vi "PhaseSpace.vi"() -> ()   [LabVIEW 2018]
uses:
  <vilib>/Platform/TimedLoop/XDataNode/timing_clust.ctl
  <vilib>/Platform/TimedLoop/XDataNode/nitl_modes.ctl
  <vilib>/Platform/TimedLoop/XDataNode/wakeup.ctl
  Global Variables/Sensor_Impluse.vi
  Global Variables/Sensor_Force.vi
  <vilib>/express/express shared/transition.llb/Dynamic To Waveform Array.vi
  <vilib>/express/express signal manip/GetorSetDDTAttributes/Set DDT Attributes/SetT0.vi
  <vilib>/express/express shared/transition.llb/Waveform Array To Dynamic.vi
  <vilib>/Platform/TimedLoop/XDataNode/XDataNode.xnode
  <vilib>/express/express signal manip/GetorSetDDTAttributes/Set DDT Attributes/Set DDT Properties.xnode
  <vilib>/Platform/TimedLoop/XDataNode/XDNodeRunTimeDep.lvlib
  <vilib>/Analysis/NI_AALBase.lvlib
  <vilib>/Analysis/NI_AALPro.lvlib
  <vilib>/Analysis/coordinate.llb/Euler Rotation Order.ctl
  <vilib>/Analysis/baseanly.llb/Real A x B.vi
  <vilib>/Analysis/baseanly.llb/A x Vector.vi
panel:
  out "A x Vector":dbl[](array[numeric]) format="%.2f"
  out "Root canal 2":dbl[](array[numeric])
  out "Count":u32
  out "element":i32
  in  "Record":bool
  in  "Save?":bool
  out "Frame 2":string
  out "LED ID":i32
  out "Y position (mm) 8":string
  out "X position (mm) 8":string
  out "Z position (mm) 8":string
  out "_LED 1":dbl[](array[numeric])
  out "Y position (mm) 9":string
  out "X position (mm) 9":string
  out "Z position (mm) 9":string
  out "_LED 2":dbl[](array[numeric])
  out "Y position (mm) 10":string
  out "X position (mm) 10":string
  out "Z position (mm) 10":string
  out "_LED3":dbl[](array[numeric])
  out "Z position (mm) 11":string
  out "Y position (mm) 11":string
  out "X position (mm) 11":string
  out "_LED4":dbl[](array[numeric])
  in  "TrackingLED 3":i32=15
  in  "TrackingLED 2":i32=15
  in  "TrackingLED 1":i32=15
  in  "Server IP address 2":string="192.168.50.40"
  in  "stop":bool
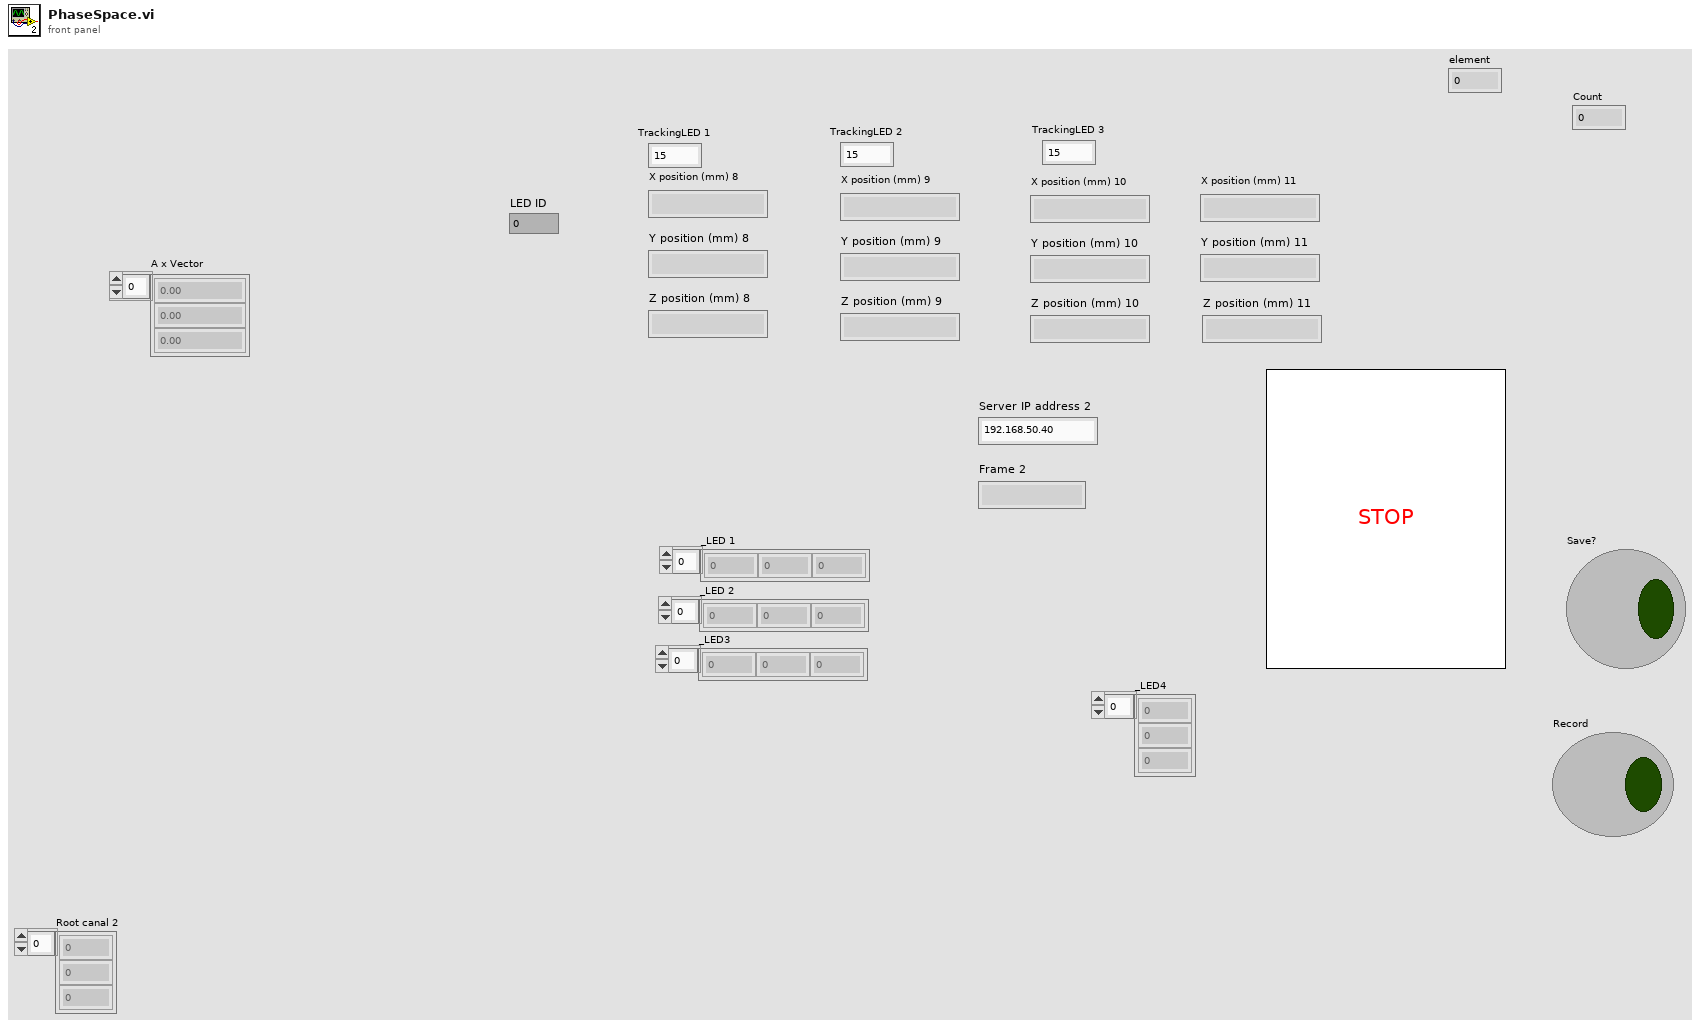
[diagram p1: front panel]
types:
  T1 = typedef "XDNodeRunTimeDep.lvlib/timing_clust.ctl" = cluster{"Expected End [f-1]":u64, "Actual End [f-1]":u64, "Finished Late? [f-1]":bool, "Expected End [i-1]":u64, "Actual End [i-1]":u64, "Finished Late? [i-1]":bool, "Expected Start [i]":u64, "Actual Start [i]":u64, "Expected Start [f]":u64, "Actual Start [f]":u64, "Source Name":string, "Structure Name":string, "Period":i64, "Deadline":i64, "Offset":i64, "Start":i64, "Priority":i32, "Timeout":i32, "Mode":T2, "Wakeup Reason":T3, "Error":errorcluster, "Source Type":string, "Secondary Source Type":string, "Global End Time":u64, "Global Start Time":u64, "Frame Duration":u64, "Iteration Duration":u64, "Assigned CPU":i32, "I/O Scan Engine Mode":u32}
  T2 = typedef "XDNodeRunTimeDep.lvlib/nitl_modes.ctl" = enum32{"No Change", "Process missed periods, maintain original phase", "Discard missed periods, maintain original phase", "Process missed periods, ignore original phase", "Discard missed periods, ignore original phase"}
  T3 = typedef "XDNodeRunTimeDep.lvlib/wakeup.ctl" = enum32{"Normal", "Aborted", "Asynchronous wakeup", "Timing source error", "Timed loop error", "Timeout"}
  T4 = typedef "NI_AALPro.lvlib/Euler Rotation Order.ctl" = u16
  T5 = typedef "NI_Matrix.lvlib/RealMatrix.ctl" = dbl[][]
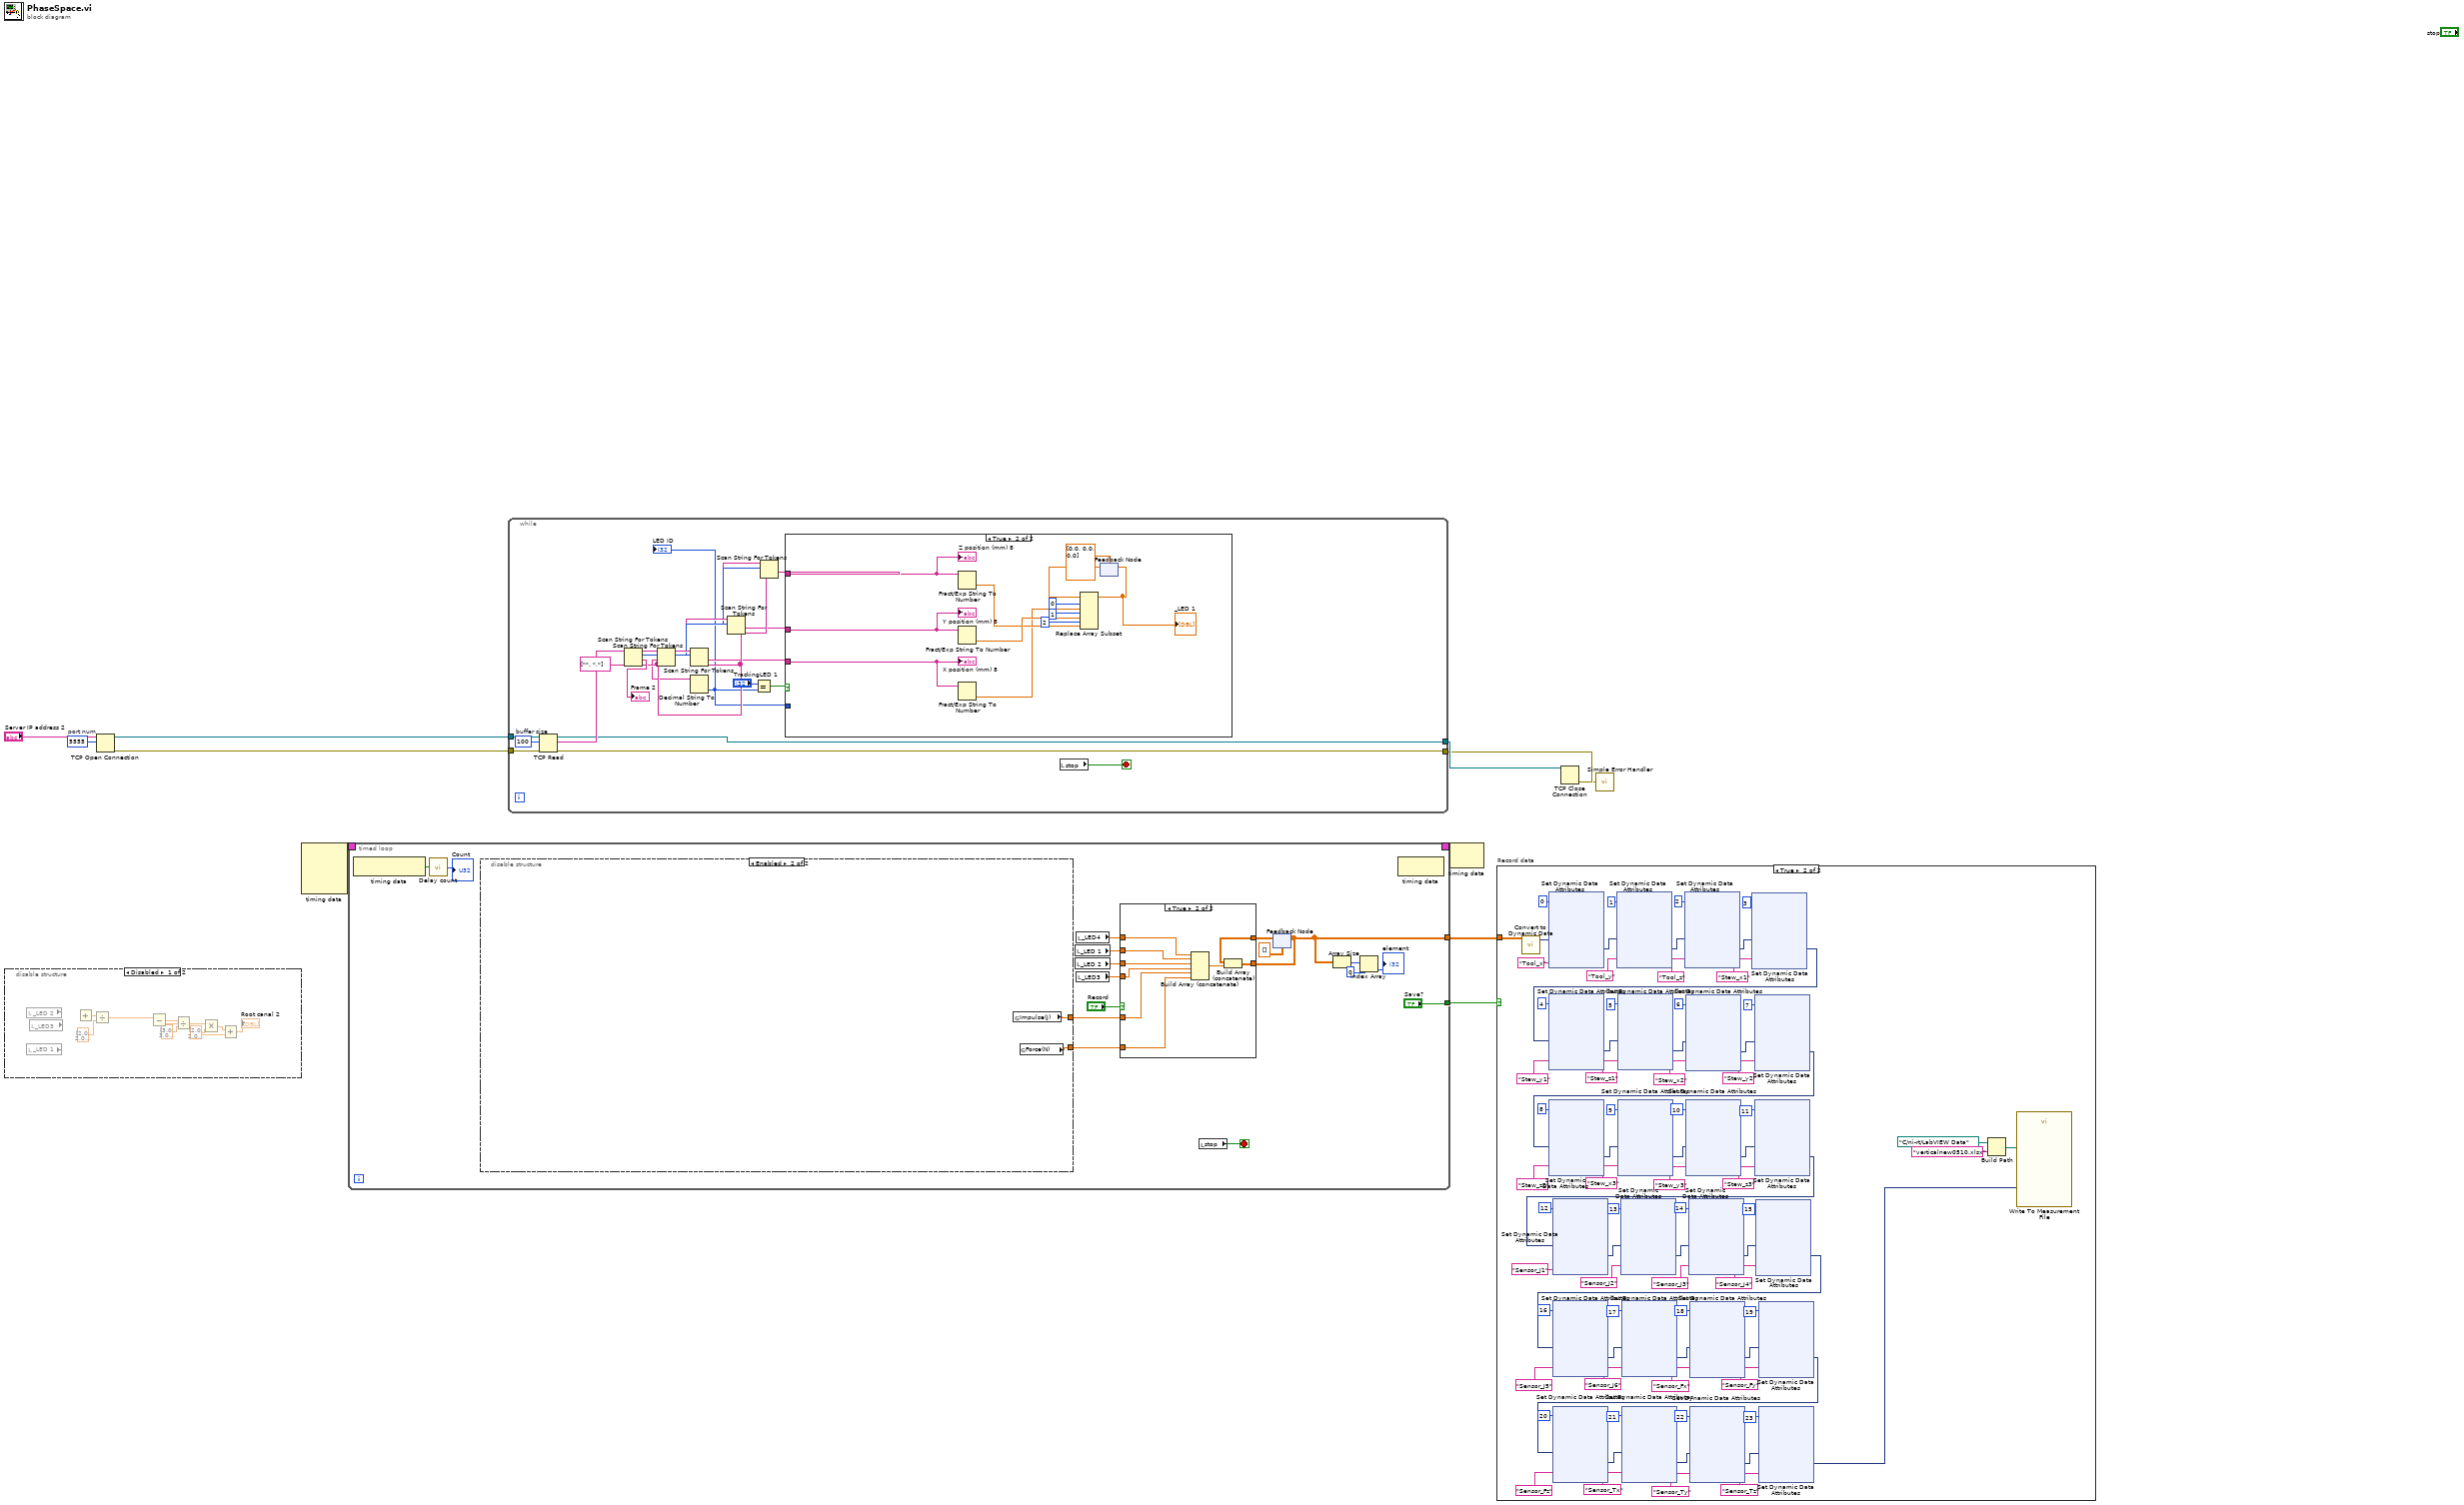
[diagram p0: block diagram]
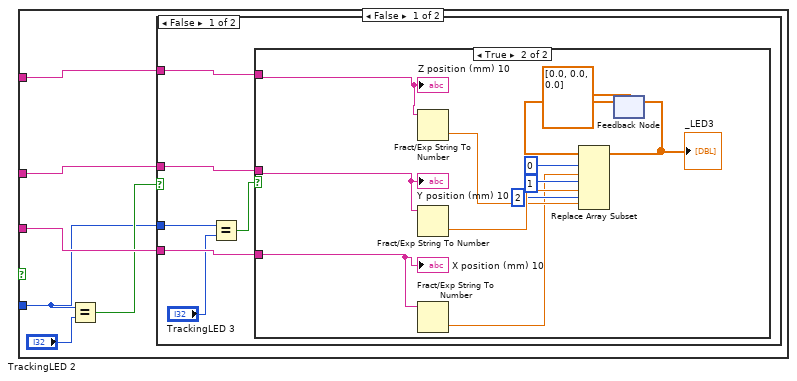
[diagram p3: hidden frame]
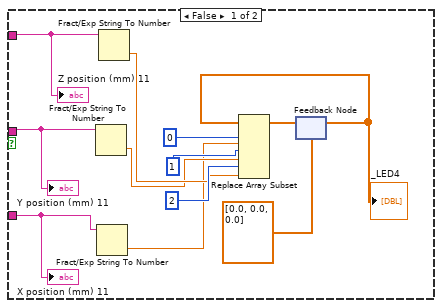
[diagram p4: hidden frame]
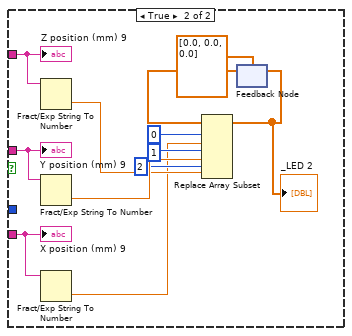
[diagram p5: hidden frame]
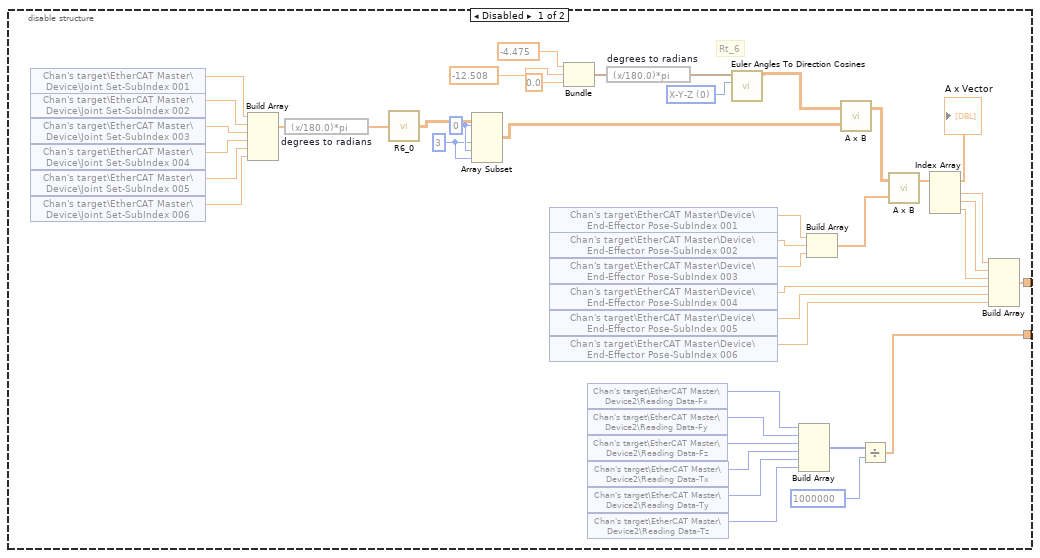
[diagram p6: hidden frame]
diagram:
  w9 = 5555  # port num
  n1 = disable-structure shown="Disabled" {
    frame Disabled {
      n2 = local read "_LED 2"() -> (w13:dbl[])
      n3 = local read "_LED 1"() -> (w12:dbl[])
      n4 = local read "_LED3"() -> ()  [unwired: 1 out]
      n5 = Add() -> (x+y=w22:dbl)  [unwired: 2 in]
      n6 = Divide(x=w22, y=dbl[] [2.0, 2.0, 2.0]) -> (x/y=w21:dbl[])
      n7 = Subtract(x=w21, y=w17) -> (x-y=w19:dbl[])
      n8 = Divide(x=w19, y=dbl[] [3.0, 3.0, 3.0]) -> (x/y=w20:dbl[])
      n9 = Multiply(x=w20, y=dbl[] [2.0, 2.0, 2.0]) -> (x*y=w18:dbl[])
      n10 = Add(x=w18) -> (y=w17:dbl[], x+y=→"Root canal 2":dbl[])
    }
    frame Enabled {
    }
  }
  n11 = TCP Open Connection(address="Server IP address 2", remote port or service name=w9) -> (connection ID=w10:refnum<k5>, error out=w11:errorcluster)  [unwired: 3 in]
  n12 = node-c288() -> (w4:T1)  [unwired: 4 in]
  n13 = timed-loop {
    timing: w4 -> [_]
    timing-out: [_] -> w3
    tunnel: ["Save?"] -> w2
    tunnel: [w35] -> w1
    stop <- w31 stop-if-true
    n14 = node-c288() -> (w30:bool)  [unwired: 1 in]
    n15 = call "Delay count.vi"("Finished Late? [i-1]"=w30) -> ("Count"=→"Count":u32)
    n16 = disable-structure shown="Enabled" {
      disable-tunnel: [w70 w83] -> w27
      disable-tunnel: [w69 w82] -> w26
      frame Disabled {
        w45 = 0 ("row 1")
        w44 = 3 ("row N")
        w52 = T4 0 items=["X-Y-Z", "X-Z-Y", "Y-X-Z", "Y-Z-X", "Z-X-Y", "Z-Y-X", "X-Y-X", "X-Z-X", "Y-X-Y", "Y-Z-Y", "Z-X-Z", "Z-Y-Z"] ("rotation order")
        # "Rt_6"
        n17 = shared-variable "Chan's target\\EtherCAT Master\\Device\\Joint Set-SubIndex 001"() -> (w68:sgl)  [unwired: 1 in, 1 out]
        n18 = shared-variable "Chan's target\\EtherCAT Master\\Device\\Joint Set-SubIndex 002"() -> (w67:sgl)  [unwired: 1 in, 1 out]
        n19 = shared-variable "Chan's target\\EtherCAT Master\\Device\\Joint Set-SubIndex 003"() -> (w66:sgl)  [unwired: 1 in, 1 out]
        n20 = shared-variable "Chan's target\\EtherCAT Master\\Device\\Joint Set-SubIndex 004"() -> (w65:sgl)  [unwired: 1 in, 1 out]
        n21 = shared-variable "Chan's target\\EtherCAT Master\\Device\\Joint Set-SubIndex 005"() -> (w64:sgl)  [unwired: 1 in, 1 out]
        n22 = shared-variable "Chan's target\\EtherCAT Master\\Device\\Joint Set-SubIndex 006"() -> (w63:sgl)  [unwired: 1 in, 1 out]
        n23 = Build Array(w68, w67, w66, w65, w64, w63) -> (w42:sgl[])
        n24 = expression code="(x/180.0)*pi" "degrees to radians"(w42) -> (w41:sgl[])
        n25 = call "R6_0.vi"("input variable"=w41) -> ("output variable"=w46:dbl[][])
        n26 = Array Subset(array=w46, index (row)=w45, length (row)=w44, index (col)=w45, length (col)=w44) -> (w43:dbl[][])
        n27 = shared-variable "Chan's target\\EtherCAT Master\\Device\\End-Effector Pose-SubIndex 001"() -> (w62:sgl)  [unwired: 1 in, 1 out]
        n28 = shared-variable "Chan's target\\EtherCAT Master\\Device\\End-Effector Pose-SubIndex 002"() -> (w61:sgl)  [unwired: 1 in, 1 out]
        n29 = shared-variable "Chan's target\\EtherCAT Master\\Device\\End-Effector Pose-SubIndex 003"() -> (w60:sgl)  [unwired: 1 in, 1 out]
        n30 = shared-variable "Chan's target\\EtherCAT Master\\Device\\End-Effector Pose-SubIndex 004"() -> (w73:sgl)  [unwired: 1 in, 1 out]
        n31 = shared-variable "Chan's target\\EtherCAT Master\\Device\\End-Effector Pose-SubIndex 005"() -> (w72:sgl)  [unwired: 1 in, 1 out]
        n32 = shared-variable "Chan's target\\EtherCAT Master\\Device\\End-Effector Pose-SubIndex 006"() -> (w71:sgl)  [unwired: 1 in, 1 out]
        n33 = Bundle("alpha"=-4.475, "alpha"=-12.508, sgl 0.0) -> (w51:cluster{"alpha":dbl, "alpha":dbl, sgl})  [unwired: 1 in]
        n34 = shared-variable "Chan's target\\EtherCAT Master\\Device2\\Reading Data-Fx"() -> (w81:i32)  [unwired: 1 in, 1 out]
        n35 = shared-variable "Chan's target\\EtherCAT Master\\Device2\\Reading Data-Fy"() -> (w80:i32)  [unwired: 1 in, 1 out]
        n36 = shared-variable "Chan's target\\EtherCAT Master\\Device2\\Reading Data-Fz"() -> (w76:i32)  [unwired: 1 in, 1 out]
        n37 = shared-variable "Chan's target\\EtherCAT Master\\Device2\\Reading Data-Tx"() -> (w79:i32)  [unwired: 1 in, 1 out]
        n38 = shared-variable "Chan's target\\EtherCAT Master\\Device2\\Reading Data-Ty"() -> (w77:i32)  [unwired: 1 in, 1 out]
        n39 = shared-variable "Chan's target\\EtherCAT Master\\Device2\\Reading Data-Tz"() -> (w78:i32)  [unwired: 1 in, 1 out]
        n40 = expression code="(x/180.0)*pi" "degrees to radians"(w51) -> (w50:cluster{"alpha":dbl, "alpha":dbl, sgl})
        n41 = call <vilib>:"Euler Angles To Direction Cosines.vi"("rotation order"=w52, "Euler Angles"=w50) -> ("Direction Cosines"=w49:dbl[][])  [unwired: 8 in, 1 out]
        n42 = Build Array(w81, w80, w76, w79, w77, w78) -> (w75:i32[])
        n43 = Build Array(w62, w61, w60) -> (w58:sgl[])
        n44 = call-poly <vilib>:"A x B.vi"("B"=w43, "A"=w49) -> ("A x B"=w59:T5)  [unwired: 1 out]
        n45 = Divide(x=w75, y=1000000) -> (x/y=w69:dbl[])
        n46 = call-poly <vilib>:"A x B.vi"("Vector"=w58, "A"=w59) -> ("A x Vector"=w57:dbl[])  [unwired: 1 out]
        "A x Vector" <- w57
        n47 = Index Array(array=w57) -> (element #1=w56:dbl, element #2=w55:dbl, element #3=w54:dbl)  [unwired: 3 in]
        n48 = Build Array(w56, w55, w54, w73, w72, w71) -> (w70:dbl[])
      }
      frame Enabled {
        n49 = global read "Sensor_Impluse.vi" "Impulse(J)"() -> (w83:dbl[])
        n50 = global read "Sensor_Force.vi" "Force(N)"() -> (w82:dbl[])
      }
    }
    n51 = local read "_LED 1"() -> (w34:dbl[])
    n52 = local read "_LED 2"() -> (w32:dbl[])
    n53 = local read "_LED4"() -> (w28:dbl[])
    n54 = local read "_LED3"() -> (w33:dbl[])
    n55 = local read "stop"() -> (w31:bool)
    n56 = feedback #1(dbl[][] []) -> (w24:dbl[][])
    n57 = case shown="True" "Record" {
      tunnel: [w84 w92] -> w35
      tunnel: w24 -> [w84 w91]
      tunnel: w32 -> [_ w88]
      tunnel: w33 -> [_ w87]
      tunnel: w34 -> [_ w89]
      tunnel: w28 -> [_ w90]
      tunnel: w27 -> [_ w86]
      tunnel: w26 -> [_ w85]
      frame False {
      }
      frame True {
        n58 = Build Array (concatenate)(w90, w89, w88, w87, w86, w85) -> (w93:dbl[])
        n59 = Build Array (concatenate)(w91, w93) -> (w92:dbl[][])
      }
    }
    n60 = feedback-in #1(w35) -> ()
    n61 = Array Size(array=w35) -> (size(s)=w38:i32[])
    n62 = Index Array(array=w38, index=0) -> (element=→"element":i32)
    n63 = node-c288() -> ()  [unwired: 1 in, 1 out]
  }
  n64 = while {
    tunnel: w10 -> [w105]
    tunnel: w11 -> [w103]
    tunnel: [w100] -> w8
    tunnel: [w102] -> w7
    stop <- w106 stop-if-true
    w115 = string[] ["", ","]
    w104 = 100  # buffer size
    n65 = TCP Read(connection ID=w105, bytes to read=w104, error in (no error)=w103) -> (connection ID out=w100:refnum<k5>, data out=w101:string, error out=w102:errorcluster)  [unwired: 2 in]
    n66 = Scan String For Tokens(6:w115, 9:w101) -> (1:→"Frame 2":string, 2:w118:i32, 3:w119:string)  [unwired: 4 in, 1 out]
    n67 = Scan String For Tokens(6:w115, 8:w118, 9:w119) -> (1:w110:string, 2:w116:i32, 3:w117:string)  [unwired: 3 in, 1 out]
    n68 = Scan String For Tokens(6:w115, 8:w116, 9:w117) -> (1:w109:string, 2:w114:i32, 3:w113:string)  [unwired: 3 in, 1 out]
    n69 = Decimal String To Number(string=w110) -> (number=w97:i32)  [unwired: 2 in, 1 out]
    "LED ID" <- w97
    n70 = Scan String For Tokens(6:w115, 8:w114, 9:w113) -> (1:w108:string, 2:w112:i32, 3:w111:string)  [unwired: 3 in, 1 out]
    n71 = Equal?(x="TrackingLED 1", y=w97) -> (x = y?=w99:bool)
    n72 = Scan String For Tokens(6:w115, 8:w112, 9:w111) -> (1:w107:string)  [unwired: 3 in, 3 out]
    n73 = case shown="True" w99 {
      tunnel: w109 -> [w124 w180]
      tunnel: w108 -> [w125 w179]
      tunnel: w107 -> [w126 w178]
      tunnel: w97 -> [w121 _]
      frame False {
        n74 = Equal?(x=w121, y="TrackingLED 2") -> (x = y?=w122:bool)
        n75 = case shown="False" w122 {
          tunnel: w126 -> [w130 w160]
          tunnel: w125 -> [w131 w159]
          tunnel: w124 -> [w132 w158]
          tunnel: w121 -> [w128 _]
          frame False {
            n76 = Equal?(x=w128, y="TrackingLED 3") -> (x = y?=w129:bool)
            n77 = case shown="True" w129 {
              tunnel: w132 -> [w142 w148]
              tunnel: w131 -> [w143 w147]
              tunnel: w130 -> [w144 w146]
              frame False {
                n78 = Fract/Exp String To Number(string=w143) -> (number=w137:dbl)  [unwired: 3 in, 1 out]
                n79 = Fract/Exp String To Number(string=w142) -> (number=w136:dbl)  [unwired: 3 in, 1 out]
                n80 = Fract/Exp String To Number(string=w144) -> (number=w138:dbl)  [unwired: 3 in, 1 out]
                n81 = feedback #2(dbl[] [0.0, 0.0, 0.0]) -> (w133:dbl[])
                "_LED4" <- w133
                n82 = Replace Array Subset(array=w133, new element #1=w136, index #1=0 ("index"), new element #2=w137, index #2=1 ("index"), new element #3=w138, index #3=2 ("index")) -> (w135:dbl[])
                n83 = feedback-in #2(w135) -> ()
                "Z position (mm) 11" <- w144
                "Y position (mm) 11" <- w143
                "X position (mm) 11" <- w142
              }
              frame True {
                n84 = Fract/Exp String To Number(string=w146) -> (number=w151:dbl)  [unwired: 3 in, 1 out]
                n85 = Fract/Exp String To Number(string=w147) -> (number=w153:dbl)  [unwired: 3 in, 1 out]
                n86 = Fract/Exp String To Number(string=w148) -> (number=w150:dbl)  [unwired: 3 in, 1 out]
                n87 = feedback #3(dbl[] [0.0, 0.0, 0.0]) -> (w156:dbl[])
                n88 = Replace Array Subset(array=w156, new element #1=w150, index #1=0 ("index"), new element #2=w153, index #2=1 ("index"), new element #3=w151, index #3=2 ("index")) -> (w145:dbl[])
                "_LED3" <- w145
                n89 = feedback-in #3(w145) -> ()
                "Y position (mm) 10" <- w147
                "X position (mm) 10" <- w148
                "Z position (mm) 10" <- w146
              }
            }
          }
          frame True {
            n90 = Fract/Exp String To Number(string=w160) -> (number=w163:dbl)  [unwired: 3 in, 1 out]
            n91 = Fract/Exp String To Number(string=w159) -> (number=w165:dbl)  [unwired: 3 in, 1 out]
            n92 = Fract/Exp String To Number(string=w158) -> (number=w162:dbl)  [unwired: 3 in, 1 out]
            n93 = feedback #4(dbl[] [0.0, 0.0, 0.0]) -> (w168:dbl[])
            n94 = Replace Array Subset(array=w168, new element #1=w162, index #1=0 ("index"), new element #2=w165, index #2=1 ("index"), new element #3=w163, index #3=2 ("index")) -> (w157:dbl[])
            "_LED 2" <- w157
            n95 = feedback-in #4(w157) -> ()
            "Y position (mm) 9" <- w159
            "X position (mm) 9" <- w158
            "Z position (mm) 9" <- w160
          }
        }
      }
      frame True {
        n96 = Fract/Exp String To Number(string=w178) -> (number=w171:dbl)  [unwired: 3 in, 1 out]
        n97 = Fract/Exp String To Number(string=w179) -> (number=w173:dbl)  [unwired: 3 in, 1 out]
        n98 = Fract/Exp String To Number(string=w180) -> (number=w170:dbl)  [unwired: 3 in, 1 out]
        n99 = feedback #5(dbl[] [0.0, 0.0, 0.0]) -> (w176:dbl[])
        n100 = Replace Array Subset(array=w176, new element #1=w170, index #1=0 ("index"), new element #2=w173, index #2=1 ("index"), new element #3=w171, index #3=2 ("index")) -> (w169:dbl[])
        "_LED 1" <- w169
        n101 = feedback-in #5(w169) -> ()
        "Y position (mm) 8" <- w179
        "X position (mm) 8" <- w180
        "Z position (mm) 8" <- w178
      }
    }
    n102 = local read "stop"() -> (w106:bool)
  }
  n103 = node-c288(w3) -> ()  [unwired: 1 out]
  n104 = case "Record data" shown="True" w2 {
    tunnel: w1 -> [_ w236]
    frame False {
    }
    frame True {
      n105 = call "Convert to Dynamic Data"("2D Array"=w236) -> ("Dynamic Data Type"=w238:dynamicdata)  [unwired: 3 in]
      n106 = xnode "Set Dynamic Data Attributes"("Signals In"=w238, "Signal Name"="Tool_x", "Signal Index"=0) -> ("Signals Out"=w240:dynamicdata)  [unwired: 1 in, 1 out]
      n107 = xnode "Set Dynamic Data Attributes"("Signals In"=w240, "Signal Name"="Tool_y", "Signal Index"=1) -> ("Signals Out"=w245:dynamicdata)  [unwired: 1 in, 1 out]
      n108 = xnode "Set Dynamic Data Attributes"("Signals In"=w245, "Signal Name"="Tool_z", "Signal Index"=2) -> ("Signals Out"=w254:dynamicdata)  [unwired: 1 in, 1 out]
      n109 = xnode "Set Dynamic Data Attributes"("Signals In"=w254, "Signal Name"="Stew_x1", "Signal Index"=3) -> ("Signals Out"=w250:dynamicdata)  [unwired: 1 in, 1 out]
      n110 = xnode "Set Dynamic Data Attributes"("Signals In"=w250, "Signal Name"="Stew_y1", "Signal Index"=4) -> ("Signals Out"=w253:dynamicdata)  [unwired: 1 in, 1 out]
      n111 = xnode "Set Dynamic Data Attributes"("Signals In"=w253, "Signal Name"="Stew_z1", "Signal Index"=5) -> ("Signals Out"=w220:dynamicdata)  [unwired: 1 in, 1 out]
      n112 = xnode "Set Dynamic Data Attributes"("Signals In"=w220, "Signal Name"="Stew_x2", "Signal Index"=6) -> ("Signals Out"=w231:dynamicdata)  [unwired: 1 in, 1 out]
      n113 = xnode "Set Dynamic Data Attributes"("Signals In"=w231, "Signal Name"="Stew_y2", "Signal Index"=7) -> ("Signals Out"=w219:dynamicdata)  [unwired: 1 in, 1 out]
      n114 = xnode "Set Dynamic Data Attributes"("Signals In"=w219, "Signal Name"="Stew_z2", "Signal Index"=8) -> ("Signals Out"=w221:dynamicdata)  [unwired: 1 in, 1 out]
      n115 = xnode "Set Dynamic Data Attributes"("Signals In"=w221, "Signal Name"="Stew_x3", "Signal Index"=9) -> ("Signals Out"=w218:dynamicdata)  [unwired: 1 in, 1 out]
      n116 = xnode "Set Dynamic Data Attributes"("Signals In"=w218, "Signal Name"="Stew_y3", "Signal Index"=10) -> ("Signals Out"=w230:dynamicdata)  [unwired: 1 in, 1 out]
      n117 = xnode "Set Dynamic Data Attributes"("Signals In"=w230, "Signal Name"="Stew_z3", "Signal Index"=11) -> ("Signals Out"=w182:dynamicdata)  [unwired: 1 in, 1 out]
      n118 = xnode "Set Dynamic Data Attributes"("Signals In"=w182, "Signal Name"="Sensor_J1", "Signal Index"=12) -> ("Signals Out"=w197:dynamicdata)  [unwired: 1 in, 1 out]
      n119 = xnode "Set Dynamic Data Attributes"("Signals In"=w197, "Signal Name"="Sensor_J2", "Signal Index"=13) -> ("Signals Out"=w192:dynamicdata)  [unwired: 1 in, 1 out]
      n120 = xnode "Set Dynamic Data Attributes"("Signals In"=w192, "Signal Name"="Sensor_J3", "Signal Index"=14) -> ("Signals Out"=w183:dynamicdata)  [unwired: 1 in, 1 out]
      n121 = xnode "Set Dynamic Data Attributes"("Signals In"=w183, "Signal Name"="Sensor_J4", "Signal Index"=15) -> ("Signals Out"=w187:dynamicdata)  [unwired: 1 in, 1 out]
      n122 = xnode "Set Dynamic Data Attributes"("Signals In"=w187, "Signal Name"="Sensor_J5", "Signal Index"=16) -> ("Signals Out"=w184:dynamicdata)  [unwired: 1 in, 1 out]
      n123 = xnode "Set Dynamic Data Attributes"("Signals In"=w184, "Signal Name"="Sensor_J6", "Signal Index"=17) -> ("Signals Out"=w215:dynamicdata)  [unwired: 1 in, 1 out]
      n124 = xnode "Set Dynamic Data Attributes"("Signals In"=w215, "Signal Name"="Sensor_Fx", "Signal Index"=18) -> ("Signals Out"=w204:dynamicdata)  [unwired: 1 in, 1 out]
      n125 = xnode "Set Dynamic Data Attributes"("Signals In"=w204, "Signal Name"="Sensor_Fy", "Signal Index"=19) -> ("Signals Out"=w216:dynamicdata)  [unwired: 1 in, 1 out]
      n126 = xnode "Set Dynamic Data Attributes"("Signals In"=w216, "Signal Name"="Sensor_Fz", "Signal Index"=20) -> ("Signals Out"=w214:dynamicdata)  [unwired: 1 in, 1 out]
      n127 = xnode "Set Dynamic Data Attributes"("Signals In"=w214, "Signal Name"="Sensor_Tx", "Signal Index"=21) -> ("Signals Out"=w217:dynamicdata)  [unwired: 1 in, 1 out]
      n128 = xnode "Set Dynamic Data Attributes"("Signals In"=w217, "Signal Name"="Sensor_Ty", "Signal Index"=22) -> ("Signals Out"=w205:dynamicdata)  [unwired: 1 in, 1 out]
      n129 = xnode "Set Dynamic Data Attributes"("Signals In"=w205, "Signal Name"="Sensor_Tz", "Signal Index"=23) -> ("Signals Out"=w181:dynamicdata)  [unwired: 1 in, 1 out]
      n130 = Build Path(base path=path "C:/ni-rt/LabVIEW Data", name or relative path="verticalnew0510.xlsx") -> (appended path=w257:path)
      n131 = call "Write To Measurement File"("Signals"=w181, "Filename"=w257) -> ()  [unwired: 15 in, 3 out]
    }
  }
  n132 = TCP Close Connection(connection ID=w8, error in (no error)=w7) -> (error out=w6:errorcluster)  [unwired: 1 in, 1 out]
  n133 = call <vilib>:"Simple Error Handler.vi"("error in (no error)"=w6) -> ()  [unwired: 2 in, 7 out]
